vi "Tower_lamp.vi"(0 "Relay_Channel_OUT":T1[](array[typedef]), 1 "FCT/EOL":bool, 5 "Modbus master in":refnum<class "Modbus Master.lvclass">, 7 "DOs":bool[](array[boolean])=[TRUE, FALSE, FALSE, FALSE], 9 "queue IN":refnum<queue>, 11 "DUT":u8) -> ()   [LabVIEW 2024, in "Relay_Module.lvlib"]
uses:
  Relay_Module.lvlib
  Relay_Enum_OUT.ctl
  <vilib>/NI/Modbus Library/API/master/Modbus Master.lvclass
  Relay_Channel_Write.ctl
panel:
  in  "queue IN 2":refnum<queue>
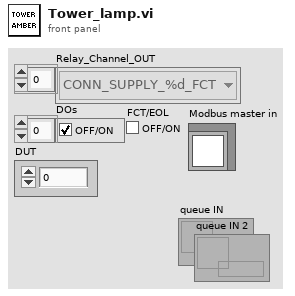
[diagram p1: front panel]
types:
  T1 = typedef "Relay_Module.lvlib/Relay_Enum_OUT.ctl" = enum16{"CONN_SUPPLY_%d_FCT", "HB_CONN_%d_FCT", "L_IND_CONN_%d_FCT", "R_IND_CONN_%d_FCT", "SW1_%d_FCT", "SW2_%d_FCT", "CAN_H_%d_FCT", "CAN_L_%d_FCT", "CYLINDER_ON/OFF_%d_FCT", "SPARE_1_%d_FCT", "SPARE_2_%d_FCT", "Tower Red", "Tower Amber", "Tower Green", "Tower Buzzer", "SLIMRELAY_DUT_%d_FCT", "GND_DMM_%d_EOL", "CAN_H_RES_%d_EOL", "CAN_L_RES_%d_EOL", "L_IND_RES_%d_EOL", "R_IND_RES_%d_EOL", "HB_CONN_DMM_%d_EOL", "14V_RES_%d_EOL", "CAN_L_(DMM-)_%d_EOL", "CAN_H_%d_EOL", "CAN_L_%d_EOL", "14V_%d_EOL", "GND_%d_EOL", "HB_CONN_%d_EOL", "L_IND_%d_EOL", "R_IND_%d_EOL", "CYLINDER_DUT_%d_EOL", "CYL_PB_1_%d_EOL", "CYL_PB_2_%d_EOL", "DUT_PASS_%d_EOL", "DUT_FAIL_%d_EOL", "SPARE1_%d_EOL", "Tower Red_EOL", "Tower Amber_EOL", "Tower Green_EOL", "Tower Buzzer_EOL"}
  T2 = typedef "Relay_Module.lvlib/Relay_Channel_Write.ctl" = cluster{"Relay_CH_Array":cluster{"On/Off":bool, "OUTPUT_Relay_Channels":T1}[]}
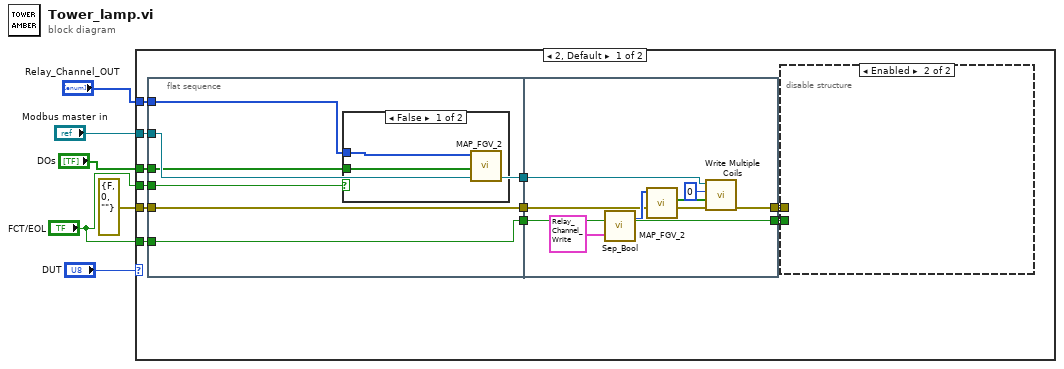
[diagram p0: block diagram]
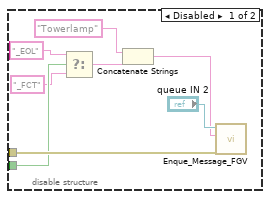
[diagram p2: hidden frame]
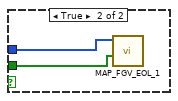
[diagram p3: hidden frame]
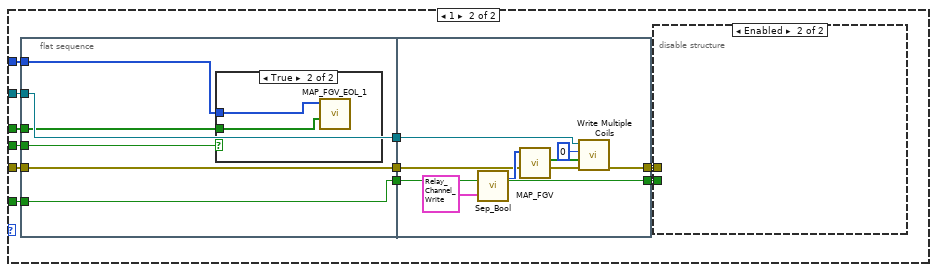
[diagram p4: hidden frame]
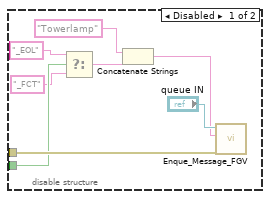
[diagram p5: hidden frame]
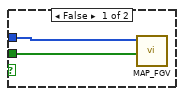
[diagram p6: hidden frame]
diagram:
  n1 = case shown="2, Default" "DUT" {
    tunnel: errorcluster {"status"=FALSE, "code"=0, "source"=""} ("error out") -> [w14 w51]
    tunnel: "Modbus master in" -> [w11 w48]
    tunnel: "DOs" -> [w10 w47]
    tunnel: "Relay_Channel_OUT" -> [w9 w46]
    tunnel: "FCT/EOL" -> [w8 w45]
    tunnel: "FCT/EOL" -> [w7 w44]
    frame 2, Default {
      n2 = flat-sequence {
        tunnel: w14 -> [w31]
        tunnel: [w31] -> w17
        tunnel: [w27] -> w16
        tunnel: [w30] -> w12
        tunnel: w11 -> [w30]
        tunnel: w10 -> [w29]
        tunnel: w9 -> [w28]
        tunnel: w8 -> [w27]
        tunnel: w7 -> [w26]
        tunnel: [w43] -> w13
        tunnel: [w37] -> w15
        tunnel: w17 -> [w38]
        tunnel: w16 -> [w43]
        tunnel: w12 -> [w36]
        frame #0 {
          n3 = case shown="False" w26 {
            tunnel: w29 -> [w33 w34]
            tunnel: w28 -> [w32 w35]
            frame False {
              n4 = call "MAP_FGV_2.vi"("DOs"=w33, "Relay_Channel_Out"=w32) -> ()  [unwired: 7 in, 3 out]
            }
            frame True {
              n5 = call "MAP_FGV_EOL_1.vi"("DOs"=w34, "Relay_Channel_Out"=w35) -> ()  [unwired: 7 in, 3 out]
            }
          }
        }
        frame #1 {
          n6 = call "Sep_Bool.vi"("output cluster"=T2 {"Relay_CH_Array"=[{"On/Off"=FALSE, "OUTPUT_Relay_Channels"=enum."CONN_SUPPLY_%d_FCT"}, {"On/Off"=FALSE, "OUTPUT_Relay_Channels"=enum."HB_CONN_%d_FCT"}, {"On/Off"=FALSE, "OUTPUT_Relay_Channels"=enum."L_IND_CONN_%d_FCT"}, {"On/Off"=FALSE, "OUTPUT_Relay_Channels"=enum."R_IND_CONN_%d_FCT"}, {"On/Off"=FALSE, "OUTPUT_Relay_Channels"=enum."SW1_%d_FCT"}, {"On/Off"=FALSE, "OUTPUT_Relay_Channels"=enum."SW2_%d_FCT"}, {"On/Off"=FALSE, "OUTPUT_Relay_Channels"=enum."CAN_H_%d_FCT"}, {"On/Off"=FALSE, "OUTPUT_Relay_Channels"=enum."CAN_L_%d_FCT"}, {"On/Off"=FALSE, "OUTPUT_Relay_Channels"=enum."CYLINDER_ON/OFF_%d_FCT"}, {"On/Off"=FALSE, "OUTPUT_Relay_Channels"=enum."SPARE_1_%d_FCT"}, {"On/Off"=FALSE, "OUTPUT_Relay_Channels"=enum."SPARE_2_%d_FCT"}, {"On/Off"=FALSE, "OUTPUT_Relay_Channels"=enum."Tower Red"}, {"On/Off"=FALSE, "OUTPUT_Relay_Channels"=enum."Tower Amber"}, {"On/Off"=FALSE, "OUTPUT_Relay_Channels"=enum."Tower Green"}, {"On/Off"=FALSE, "OUTPUT_Relay_Channels"=enum."Tower Buzzer"}, {"On/Off"=FALSE, "OUTPUT_Relay_Channels"=enum."SLIMRELAY_DUT_%d_FCT"}]} ("Relay_Channel_Write")) -> ("Array"=w41:T1[])  [unwired: 1 in, 1 out]
          n7 = call "MAP_FGV_2.vi"("Relay_Channel_Out"=w41) -> ("DOs_out"=w42:bool[])  [unwired: 8 in, 2 out]
          n8 = call-dynamic "Write Multiple Coils.vi"("error in"=w38, "coils to write"=w42, "starting address"=u16 0, "Modbus master in"=w36) -> ("error out"=w37:errorcluster)  [unwired: 6 in, 1 out]
        }
      }
      n9 = disable-structure shown="Enabled" {
        disable-tunnel: w15 -> [w25 _]
        disable-tunnel: w13 -> [w23 _]
        frame Disabled {
          n10 = Select(t="_EOL", s=w23, f="_FCT") -> (s? t:f=w22:string)
          n11 = Concatenate Strings("Towerlamp", w22) -> (w18:string)
          n12 = call "Enque_Message_FGV.vi"("error in (no error)"=w25, "Message"=w18, "queue IN"="queue IN 2") -> ()  [unwired: 8 in, 1 out]
        }
        frame Enabled {
        }
      }
    }
    frame 1 {
      n13 = flat-sequence {
        tunnel: w51 -> [w68]
        tunnel: [w68] -> w54
        tunnel: [w64] -> w53
        tunnel: [w67] -> w49
        tunnel: w48 -> [w67]
        tunnel: w47 -> [w66]
        tunnel: w46 -> [w65]
        tunnel: w45 -> [w64]
        tunnel: w44 -> [w63]
        tunnel: [w80] -> w50
        tunnel: [w74] -> w52
        tunnel: w54 -> [w75]
        tunnel: w53 -> [w80]
        tunnel: w49 -> [w73]
        frame #0 {
          n14 = case shown="True" w63 {
            tunnel: w66 -> [w70 w71]
            tunnel: w65 -> [w69 w72]
            frame False {
              n15 = call "MAP_FGV.vi"("DOs"=w70, "Relay_Channel_Out"=w69) -> ()  [unwired: 7 in, 3 out]
            }
            frame True {
              n16 = call "MAP_FGV_EOL_1.vi"("DOs"=w71, "Relay_Channel_Out"=w72) -> ()  [unwired: 7 in, 3 out]
            }
          }
        }
        frame #1 {
          n17 = call "Sep_Bool.vi"("output cluster"=T2 {"Relay_CH_Array"=[{"On/Off"=FALSE, "OUTPUT_Relay_Channels"=enum."CONN_SUPPLY_%d_FCT"}, {"On/Off"=FALSE, "OUTPUT_Relay_Channels"=enum."HB_CONN_%d_FCT"}, {"On/Off"=FALSE, "OUTPUT_Relay_Channels"=enum."L_IND_CONN_%d_FCT"}, {"On/Off"=FALSE, "OUTPUT_Relay_Channels"=enum."R_IND_CONN_%d_FCT"}, {"On/Off"=FALSE, "OUTPUT_Relay_Channels"=enum."SW1_%d_FCT"}, {"On/Off"=FALSE, "OUTPUT_Relay_Channels"=enum."SW2_%d_FCT"}, {"On/Off"=FALSE, "OUTPUT_Relay_Channels"=enum."CAN_H_%d_FCT"}, {"On/Off"=FALSE, "OUTPUT_Relay_Channels"=enum."CAN_L_%d_FCT"}, {"On/Off"=FALSE, "OUTPUT_Relay_Channels"=enum."CYLINDER_ON/OFF_%d_FCT"}, {"On/Off"=FALSE, "OUTPUT_Relay_Channels"=enum."SPARE_1_%d_FCT"}, {"On/Off"=FALSE, "OUTPUT_Relay_Channels"=enum."SPARE_2_%d_FCT"}, {"On/Off"=FALSE, "OUTPUT_Relay_Channels"=enum."Tower Red"}, {"On/Off"=FALSE, "OUTPUT_Relay_Channels"=enum."Tower Amber"}, {"On/Off"=FALSE, "OUTPUT_Relay_Channels"=enum."Tower Green"}, {"On/Off"=FALSE, "OUTPUT_Relay_Channels"=enum."Tower Buzzer"}, {"On/Off"=FALSE, "OUTPUT_Relay_Channels"=enum."SLIMRELAY_DUT_%d_FCT"}]} ("Relay_Channel_Write")) -> ("Array"=w78:T1[])  [unwired: 1 in, 1 out]
          n18 = call "MAP_FGV.vi"("Relay_Channel_Out"=w78) -> ("DOs_out"=w79:bool[])  [unwired: 8 in, 2 out]
          n19 = call-dynamic "Write Multiple Coils.vi"("error in"=w75, "coils to write"=w79, "starting address"=u16 0, "Modbus master in"=w73) -> ("error out"=w74:errorcluster)  [unwired: 6 in, 1 out]
        }
      }
      n20 = disable-structure shown="Enabled" {
        disable-tunnel: w52 -> [w62 _]
        disable-tunnel: w50 -> [w60 _]
        frame Disabled {
          n21 = Select(t="_EOL", s=w60, f="_FCT") -> (s? t:f=w59:string)
          n22 = Concatenate Strings("Towerlamp", w59) -> (w55:string)
          n23 = call "Enque_Message_FGV.vi"("error in (no error)"=w62, "Message"=w55, "queue IN"="queue IN") -> ()  [unwired: 8 in, 1 out]
        }
        frame Enabled {
        }
      }
    }
  }
